vi "getCamera.vi"(8 "error in (no error)":errorcluster, 11 "CameraTempController.lvclass in":refnum<class "CameraTempController.lvclass">) -> (0 "error out":errorcluster, 2 "Camera":enum16{"AndorIKon", "ICCamera"}(ring)=enum."ICCamera", 3 "CameraTempController.lvclass out":refnum<class "CameraTempController.lvclass">)   [LabVIEW 2011, in "Hardware.lvlib" / "Channels.lvlib" / "CameraTempController.lvclass"]
uses:
  CameraTempController.lvclass
  CameraTempController.lvclass/CameraTempController.ctl
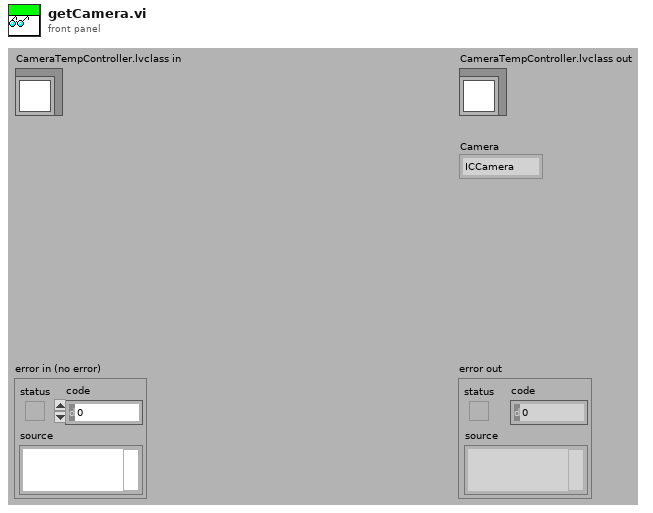
[diagram p1: front panel]
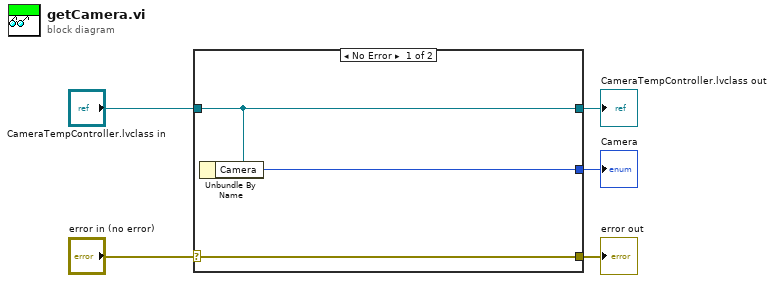
[diagram p0: block diagram]
diagram:
  n1 = case shown="No Error" "error in (no error)" {
    selector: "error in (no error)" -> [w8 w9]
    tunnel: [w8 w9] -> w4
    tunnel: [w7 w10] -> w2
    tunnel: "CameraTempController.lvclass in" -> [w7 w10]
    tunnel: [w6 _] -> w1
    frame No Error {
      n2 = Unbundle By Name(w7) -> ("Camera"=w6:enum16{"AndorIKon", "ICCamera"})
    }
    frame Error {
    }
  }
  "error out" <- w4
  "CameraTempController.lvclass out" <- w2
  "Camera" <- w1
